vi "ConfigureTestPanel.vi"(8 "error in (no error)":errorcluster) -> (0 "error out":errorcluster, 3 "Test Panel Config out":T1)   [LabVIEW 2017, in "EmsaTestPanel.lvlib"]
uses:
  <vilib>/addons/InsightCM/Devices/Shared/Emsa/EmsaTestPanel/EmsaTestPanel.lvlib
  <vilib>/addons/InsightCM/Devices/Shared/Emsa/EmsaTestPanel/controls/Configuration.ctl
  <vilib>/addons/InsightCM/Devices/Shared/Emsa/EmsaTestPanel/controls/DataSetType.ctl
  <vilib>/addons/InsightCM/Devices/Shared/Common/TestPanel/controls/Configuration.ctl
  <vilib>/addons/InsightCM/Devices/Shared/Common/TestPanel/controls/State.ctl
  <vilib>/addons/InsightCM/MessageBus/Base/controls/IRoutingSource.ctl
  <vilib>/addons/InsightCM/MessageBus/Base/controls/TestPanelTimeSeries.ctl
  <vilib>/addons/InsightCM/MessageBus/Base/controls/TestPanelValue.ctl
  <vilib>/addons/InsightCM/Utilities/GlobalConfiguration/GlobalConfiguration.lvlib
  <vilib>/addons/InsightCM/Utilities/DeviceModelHelpers/DeviceModelHelpers.lvlib
  <vilib>/addons/InsightCM/Utilities/PropertyHelpers/PropertyHelpers.lvlib
  <vilib>/addons/InsightCM/Devices/Shared/Common/TestPanel/TestPanel.lvlib
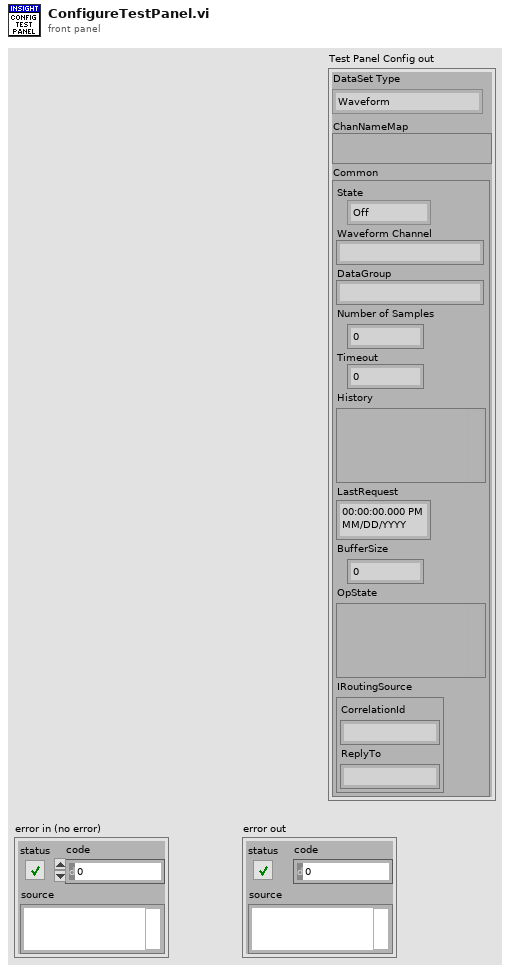
[diagram p1: front panel]
types:
  T1 = typedef "EmsaTestPanel.lvlib/Configuration.ctl" = cluster{"DataSet Type":T2, "ChanNameMap":variant, "Common":T3}
  T2 = typedef "EmsaTestPanel.lvlib/DataSetType.ctl" = enum16{"Waveform", "Sweep", "WAV"}
  T3 = typedef "TestPanel.lvlib/Configuration.ctl" = cluster{"State":T4, "Waveform Channel":string, "DataGroup":string, "Number of Samples":i32, "Timeout":dbl, "History":variant, "LastRequest":timestamp, "BufferSize":i32, "OpState":variant, "IRoutingSource":T5}
  T4 = typedef "TestPanel.lvlib/State.ctl" = enum16{"Off", "On", "PendingValues", "PendingDataSet"}
  T5 = typedef "IRoutingSource.ctl" = cluster{"CorrelationId":string, "ReplyTo":string}
  T6 = typedef "SectionKeyValues.ctl" = cluster{"Section":string, "KeyValues":T7[]}
  T7 = typedef "KeyValuePair.ctl" = cluster{"Key":string, "Value":string}
  T8 = typedef "R2_DeviceModel.ctl" = cluster{"Device":T9, "Channels":T16[], "Tags":T18[]}
  T9 = typedef "R2_Device.ctl" = cluster{"Id":string, "Name":string, "DeviceType":string, "HardwareName":string, "IpAddress":string, "HardwareInfo":T7[], "ApplicationType":string, "ApplicationVersion":string, "EquipmentIds":string[], "ConfigurationVersion":string, "State":T10, "Properties":T7[], "DataGroups":T11[], "BurstModeTrigger":T15}
  T10 = typedef "DeviceState.ctl" = cluster{"Disabled":bool}
  T11 = typedef "R2_DataGroup.ctl" = cluster{"Name":string, "OperatingStates":T12[], "Properties":T7[], "EquipmentIds":string[], "AssetNodeId":string}
  T12 = typedef "OperatingState.ctl" = cluster{"Name":string, "Properties":T7[], "Triggers":T13[]}
  T13 = typedef "Trigger.ctl" = cluster{"Type":string, "Expression":string, "Conditions":T14[]}
  T14 = typedef "Condition.ctl" = cluster{"Source":string, "Type":string, "Operator":string, "CompareTo":string, "DwellSeconds":dbl}
  T15 = typedef "BurstModeTrigger.ctl" = cluster{"Trigger":T13, "SampleRate":string, "AcquisitionLength":string}
  T16 = typedef "R2_Channel.ctl" = cluster{"Id":string, "DeviceId":string, "Name":string, "ChannelType":string, "HardwareKey":string, "HardwareChannel":string, "DataGroup":string, "Keywords":string[], "EquipmentIds":string[], "Properties":T7[], "Metrics":T17[], "AssetNodeId":string, "MeasType":string, "AssetName":string}
  T17 = typedef "Metric.ctl" = cluster{"Id":string, "Name":string, "Unit":string, "Properties":T7[], "MetricDefinitionInstanceId":string}
  T18 = typedef "Tag.ctl" = cluster{"Id":string, "Path":string, "Name":string, "Datatype":string, "Props":T7[], "Keywords":string[]}
  T19 = typedef "AssetNode.ctl" = cluster{"Id":string, "Type":string, "Name":string, "ParentIds":string[], "State":T20, "MeasType":string, "Properties":T7[], "OperatingStates":T12[], "Metrics":T17[], "TrendAlarmRules":T21[], "References":T24[]}
  T20 = typedef "AssetState.ctl" = cluster{"Disabled":bool}
  T21 = typedef "TrendAlarmRule.ctl" = cluster{"Id":string, "AssetNodeId":string, "TrendId":string, "Disabled":bool, "OperatingState":string, "Operator":string, "Hysteresis":dbl, "OnDelaySeconds":dbl, "OffDelaySeconds":dbl, "Levels":T22[], "Properties":T7[]}
  T22 = typedef "TrendAlarmLevel.ctl" = cluster{"Severity":i32, "CompareTo":dbl, "Actions":T23[]}
  T23 = typedef "AlarmAction.ctl" = cluster{"Type":string, "Props":T7[]}
  T24 = typedef "AssetNodeReference.ctl" = cluster{"NodeId":string, "Name":string}
  T25 = typedef "TestPanelTimeSeries.ctl" = cluster{"TrendPointId":string, "AssetName":string, "MetricName":string, "Unit":string, "Values":T26[]}
  T26 = typedef "TestPanelValue.ctl" = cluster{"Value":dbl, "Timestamp":i64, "Invalid":bool}
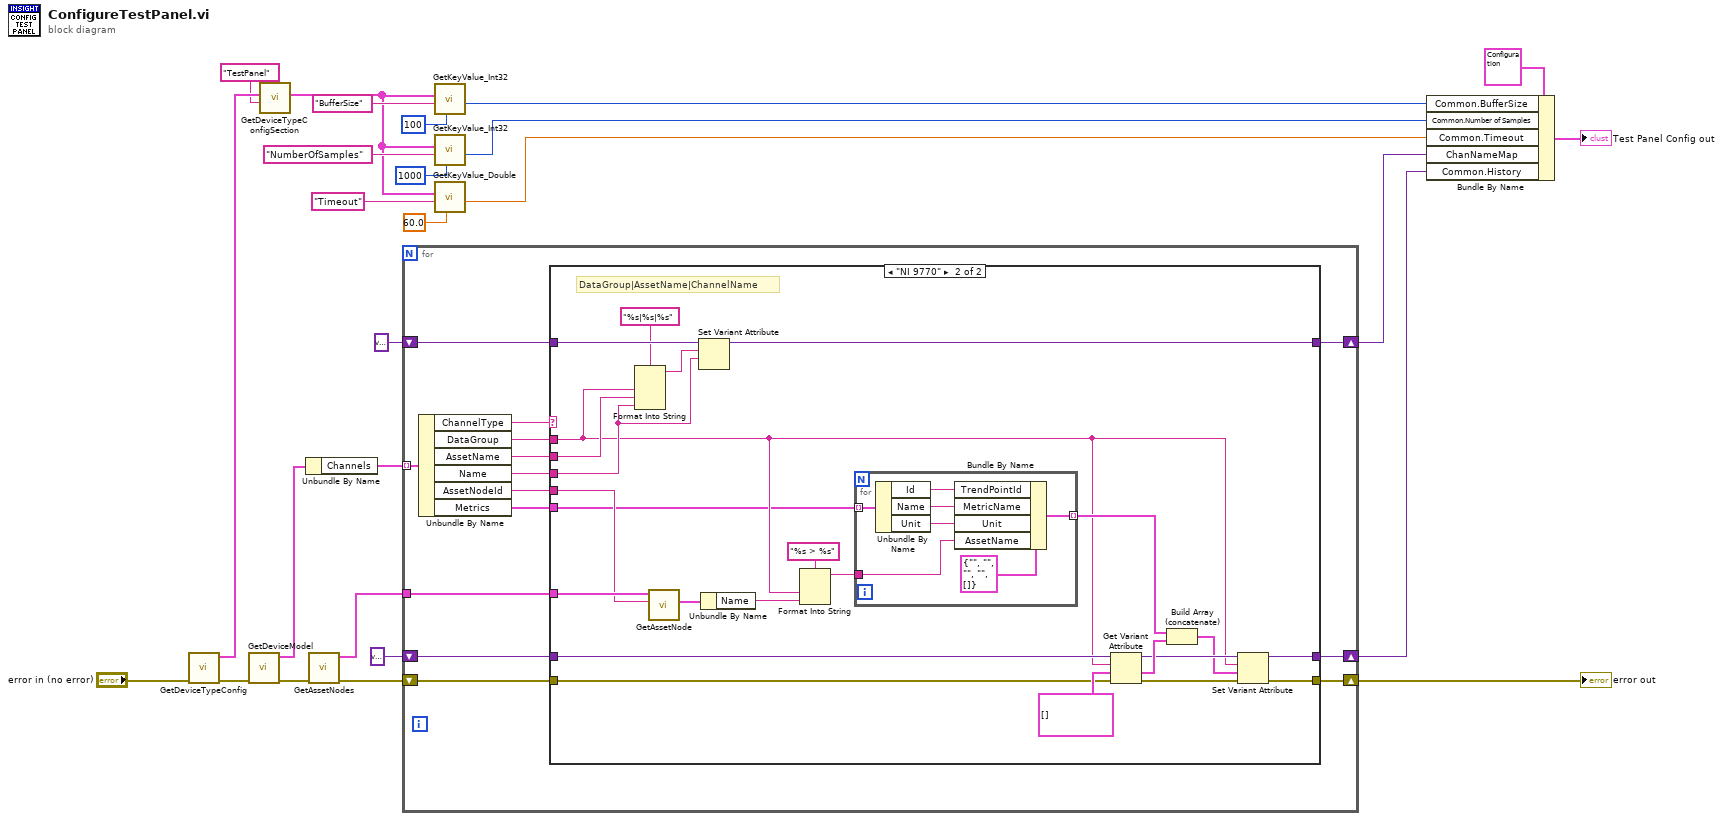
[diagram p0: block diagram]
diagram:
  n1 = call <vilib>:"GetDeviceTypeConfig.vi"("error in (no error)"="error in (no error)") -> ("error out"=w9:errorcluster, "key values"=w21:T6[])  [unwired: 8 in, 1 out]
  n2 = call <vilib>:"GetDeviceModel.vi"("error in (no error)"=w9) -> ("error out"=w10:errorcluster, "device model"=w24:T8)  [unwired: 8 in, 1 out]
  n3 = call <vilib>:"GetDeviceTypeConfigSection.vi"("key"="TestPanel", "key values"=w21) -> ("key value pairs out"=w6:T7[])  [unwired: 8 in, 1 out]
  n4 = Unbundle By Name(w24) -> ("Channels"=w3:T16[])
  n5 = call <vilib>:"GetAssetNodes.vi"("error in (no error)"=w10) -> ("error out"=w11:errorcluster, "AssetNodes"=w23:T19[])  [unwired: 8 in, 1 out]
  n6 = for {
    tunnel: w3 -> [w32] mode=indexing
    tunnel: w23 -> [w40]
    shift-right: [w37] -> w13
    shift-left: variant -> [w38]
    shift-right: [w36] -> w12
    shift-left: w11 -> [w35]
    shift-right: [w33] -> w1
    shift-left: variant -> [w34]
    n7 = Unbundle By Name(w32) -> ("ChannelType"=w28:string, "DataGroup"=w29:string, "AssetName"=w31:string, "Name"=w30:string, "AssetNodeId"=w39:string, "Metrics"=w27:T17[])
    n8 = case shown="\"NI 9770\"" w28 {
      tunnel: w40 -> [_ w67]
      tunnel: w39 -> [_ w66]
      tunnel: w38 -> [w43 w65]
      tunnel: [w43 w59] -> w37
      tunnel: [w42 w57] -> w36
      tunnel: w35 -> [w42 w56]
      tunnel: w34 -> [w41 w55]
      tunnel: [w41 w54] -> w33
      tunnel: w31 -> [_ w53]
      tunnel: w30 -> [_ w52]
      tunnel: w29 -> [_ w51]
      tunnel: w27 -> [_ w44]
      frame Default {
      }
      frame "NI 9770" {
        # "DataGroup|AssetName|ChannelName"
        n9 = Format Into String(format string="%s|%s|%s", w51, w53, w52) -> (resulting string=w45:string)  [unwired: 2 in, 1 out]
        n10 = call <vilib>:"GetAssetNode.vi"("node id"=w66, "nodes in"=w67) -> ("AssetNode"=w47:T19)  [unwired: 7 in, 2 out]
        n11 = Set Variant Attribute(Variant=w55, name=w45, value=w52) -> (Variant out=w54:variant)  [unwired: 1 in, 2 out]
        n12 = Unbundle By Name(w47) -> ("Name"=w49:string)
        n13 = Format Into String(format string="%s > %s", w51, w49) -> (resulting string=w48:string)  [unwired: 2 in, 1 out]
        n14 = for {
          tunnel: w44 -> [w73] mode=indexing
          tunnel: [w71] -> w62 mode=indexing
          tunnel: w48 -> [w68]
          n15 = Unbundle By Name(w73) -> ("Id"=w72:string, "Name"=w70:string, "Unit"=w69:string)
          n16 = Bundle By Name(cluster=T25 {"TrendPointId"="", "AssetName"="", "MetricName"="", "Unit"="", "Values"=[]} ("History"), "TrendPointId"=w72, "MetricName"=w70, "Unit"=w69, "AssetName"=w68) -> (w71:T25)
        }
        n17 = Get Variant Attribute(Variant=w65, name=w51, default value (empty Variant)=T25[] [], error in=w56) -> (duplicate Variant=w61:variant, value=w63:T25[], error out=w58:errorcluster)  [unwired: 1 out]
        n18 = Build Array (concatenate)(w62, w63) -> (w60:T25[])
        n19 = Set Variant Attribute(Variant=w61, name=w51, value=w60, error in=w58) -> (Variant out=w59:variant, error out=w57:errorcluster)  [unwired: 1 out]
      }
    }
  }
  "error out" <- w12
  n20 = call <vilib>:"GetKeyValue_Int32.vi"("default"=100, "key"="BufferSize", "key value pairs"=w6) -> ("value"=w4:i32)  [unwired: 6 in, 2 out]
  n21 = call <vilib>:"GetKeyValue_Int32.vi"("default"=1000, "key"="NumberOfSamples", "key value pairs"=w6) -> ("value"=w14:i32)  [unwired: 6 in, 2 out]
  n22 = call <vilib>:"GetKeyValue_Double.vi"("default"=60.0, "key"="Timeout", "key value pairs"=w6) -> ("value"=w15:dbl)  [unwired: 6 in, 2 out]
  n23 = Bundle By Name(cluster=T1 {"DataSet Type"=enum."Waveform", "ChanNameMap"=variant, "Common"={"State"=enum."Off", "Waveform Channel"="", "DataGroup"="", "Number of Samples"=0, "Timeout"=0.0, "History"=variant, "LastRequest"=timestamp(0 s since 1904-01-01), "BufferSize"=0, "OpState"=variant, "IRoutingSource"={"CorrelationId"="", "ReplyTo"=""}}} ("Test Panel Config"), "Common.BufferSize"=w4, "Common.Number of Samples"=w14, "Common.Timeout"=w15, "ChanNameMap"=w1, "Common.History"=w13) -> (→"Test Panel Config out":T1)
